vi "hydraharp_compute_correlation_laurence.vi"(8 "error in (no error)":errorcluster, 11 "hydraharp in":refnum<class "hydraharp.lvclass">) -> (0 "error out":errorcluster, 3 "hydraharp out":refnum<class "hydraharp.lvclass">)   [LabVIEW 2015, in "hydraharp.lvclass"]
uses:
  hydraharp.lvclass
  hydraharp.lvclass/hydraharp.ctl
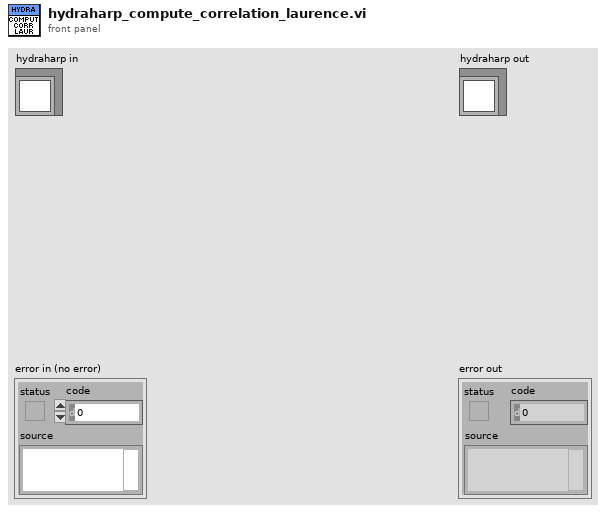
[diagram p1: front panel]
types:
  T1 = typedef "hydraharp_action_on_records.ctl" = enum16{"stream_to_file", "correlate", "stream to file and correlate", "histogram"}
  T2 = typedef "hpanel_acq_modes.ctl" = u16
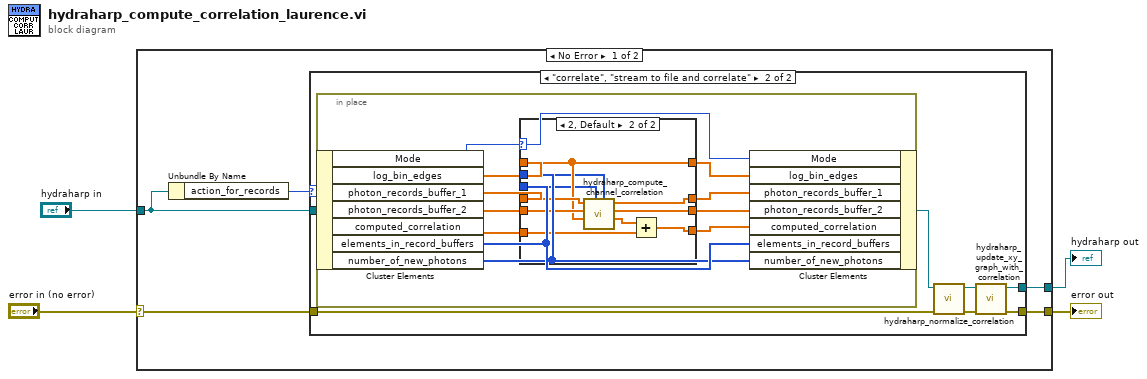
[diagram p0: block diagram]
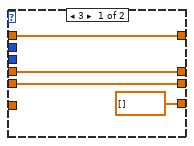
[diagram p3: hidden frame]
diagram:
  n1 = case shown="No Error" "error in (no error)" {
    selector: "error in (no error)" -> [w9 w45]
    tunnel: [w8 w45] -> w3
    tunnel: [w7 w44] -> w1
    tunnel: "hydraharp in" -> [w6 w44]
    frame No Error {
      n2 = Unbundle By Name(w6) -> ("action_for_records"=w5:T1)
      n3 = case shown="\"correlate\", \"stream to file and correlate\"" w5 {
        tunnel: w9 -> [w10 w17]
        tunnel: [w10 w13] -> w8
        tunnel: [w11 w12] -> w7
        tunnel: w6 -> [w11 w16]
        frame "stream_to_file", Default {
        }
        frame "correlate", "stream to file and correlate" {
          n4 = in-place {
            n5 = in-place-cluster #1(w16) -> ("Mode"=w28:T2, "log_bin_edges"=w29:dbl[], "photon_records_buffer_1"=w26:dbl[], "photon_records_buffer_2"=w25:dbl[], "computed_correlation"=w19:dbl[], "elements_in_record_buffers"=w21:i32[], "number_of_new_photons"=w20:i32[])
            n6 = case shown="2, Default" w28 {
              tunnel: w29 -> [w33 w39]
              tunnel: [w33 w39] -> w27
              tunnel: w26 -> [w32 w43]
              tunnel: w25 -> [w31 w42]
              tunnel: [w32 w41] -> w24
              tunnel: [w31 w40] -> w23
              tunnel: [dbl[] [] ("Corr_norm") w35] -> w22
              tunnel: w21 -> [_ w38]
              tunnel: w20 -> [_ w37]
              tunnel: w19 -> [_ w34]
              frame 3 {
              }
              frame 2, Default {
                n7 = call "hydraharp_compute_channel_correlation.vi"("number_of_new_photons"=w37, "elements_in_record_buffers"=w38, "log_bin_edges"=w39, "ch2_photons"=w42, "ch1_photons"=w43) -> ("Corr"=w36:dbl[], "ch2_photons_out"=w40:dbl[], "ch1_photons_out"=w41:dbl[])  [unwired: 4 in]
                n8 = Add(x=w36, y=w34) -> (x+y=w35:dbl[])
              }
            }
            n9 = in-place-cluster #1("Mode"=w28, "log_bin_edges"=w27, "photon_records_buffer_1"=w24, "photon_records_buffer_2"=w23, "computed_correlation"=w22, "elements_in_record_buffers"=w21, "number_of_new_photons"=w20) -> (w18:refnum<class "hydraharp.lvclass">)
          }
          n10 = call "hydraharp_normalize_correlation.vi"("error in (no error)"=w17, "hydraharp.lvclass"=w18) -> ("error out"=w14:errorcluster, "hydraharp.lvclass 2"=w15:refnum<class "hydraharp.lvclass">)  [unwired: 8 in]
          n11 = call "hydraharp_update_xy_graph_with_correlation.vi"("error in (no error)"=w14, "hydraharp in"=w15) -> ("error in (no error) 2"=w13:errorcluster, "hydraharp in 2"=w12:refnum<class "hydraharp.lvclass">)  [unwired: 8 in]
        }
      }
    }
    frame Error {
    }
  }
  "error out" <- w3
  "hydraharp out" <- w1
